vi "Ej9.vi"() -> ()   [LabVIEW 2023]
panel:
  in  "String":string
  in  "Boolean":bool
  in  "Limit":dbl format="%_3g"
  in  "stop":bool
  in  "Tank Horizontal Position":i32(slide) scale=0.0..400.0
  in  "Tank Vertical Position":i32(slide) scale=0.0..300.0
  out "Tank":dbl(slide) scale=0.0..10.0
  in  "Disable":bool
  # "True"
  # "False"
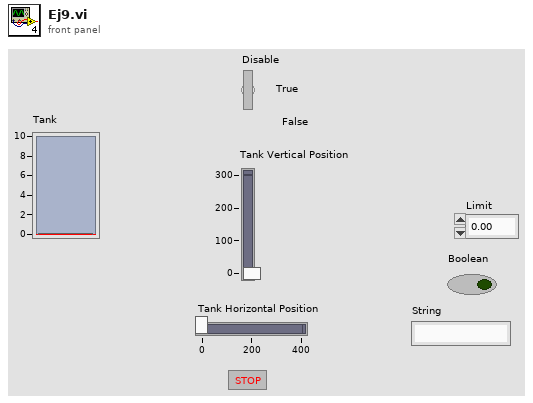
[diagram p1: front panel]
types:
  T1 = cluster{"Tank Horizontal Position":i32, "Tank Vertical Position":i32}
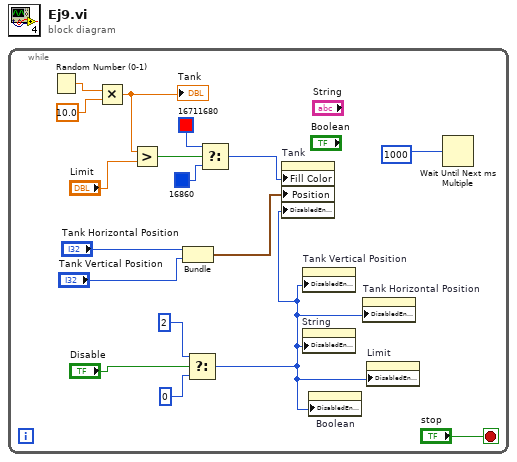
[diagram p0: block diagram]
diagram:
  n1 = while {
    stop <- "stop" stop-if-true
    n2 = Random Number (0-1)() -> (number: 0 to 1=w12:dbl)
    n3 = Multiply(x=w12, y=10.0) -> (x*y=w6:dbl)
    "Tank" <- w6
    n4 = Greater?(x=w6, y="Limit") -> (0:w9:bool)
    n5 = Bundle("Tank Horizontal Position"="Tank Horizontal Position", "Tank Vertical Position"="Tank Vertical Position") -> (w4:T1)  [unwired: 1 in]
    n6 = Select(t=2, s="Disable", f=0) -> (s? t:f=w3:i32)
    n7 = Select(t=u32 16711680, s=w9, f=u32 16860) -> (s? t:f=w5:u32)
    n8 = property on="Tank" class="Slide (strict)"("Fill Color"=w5, "Position"=w4, "DisabledEnum"=w3) -> ()  [unwired: 2 in, 2 out]
    n9 = property on="Tank Vertical Position" class="Slide (strict)"("DisabledEnum"=w3) -> ()  [unwired: 2 in, 2 out]
    n10 = property on="String" class="Str"("DisabledEnum"=w3) -> ()  [unwired: 2 in, 2 out]
    n11 = property on="Boolean" class="Bool (strict)"("DisabledEnum"=w3) -> ()  [unwired: 2 in, 2 out]
    n12 = property on="Tank Horizontal Position" class="Slide (strict)"("DisabledEnum"=w3) -> ()  [unwired: 2 in, 2 out]
    n13 = property on="Limit" class="DigNum (strict)"("DisabledEnum"=w3) -> ()  [unwired: 2 in, 2 out]
    n14 = Wait Until Next ms Multiple(millisecond multiple=1000) -> ()  [unwired: 1 out]
  }
